vi "Information.vi"(8 "error in (no error)":errorcluster, 9 "Context":T1, 10 "Information":refnum<class "Information.lvclass">, 11 "Channel Scanner in":refnum<class "Channel Scanner.lvclass">) -> (0 "error out":errorcluster, 3 "Channel Scanner out":refnum<class "Channel Scanner.lvclass">)   [LabVIEW 2021, in "Channel Scanner.lvclass"]
uses:
  Channel Scanner.lvclass
  Publish-Subscribe/Interfaces/Information/Information.lvclass
  Publish-Subscribe/Context.ctl
  NHMFL_Core/Libraries/Instruments/Results/Acquired Result/Acquired Result.lvclass
  Channel Scanner.lvclass/Channel Scanner.ctl
  Read Channel scanner configuration.vi
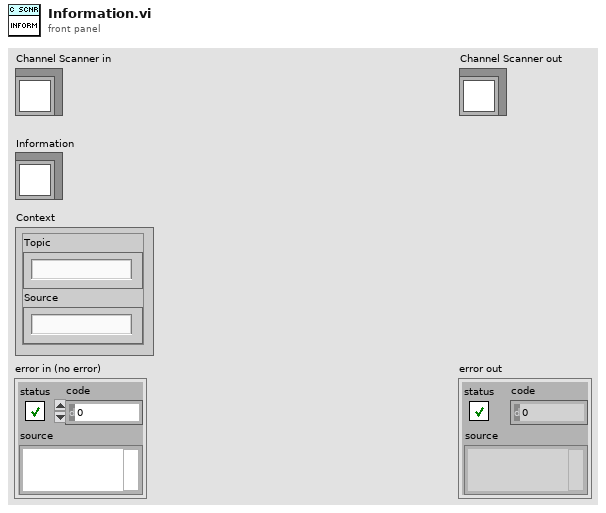
[diagram p1: front panel]
types:
  T1 = typedef "Context.ctl" = cluster{"Topic":string, "Source":string}
  T2 = typedef "Channel Scanner Configuration.ctl" = cluster{"Scan channels":i32[], "Group with measurement":string}
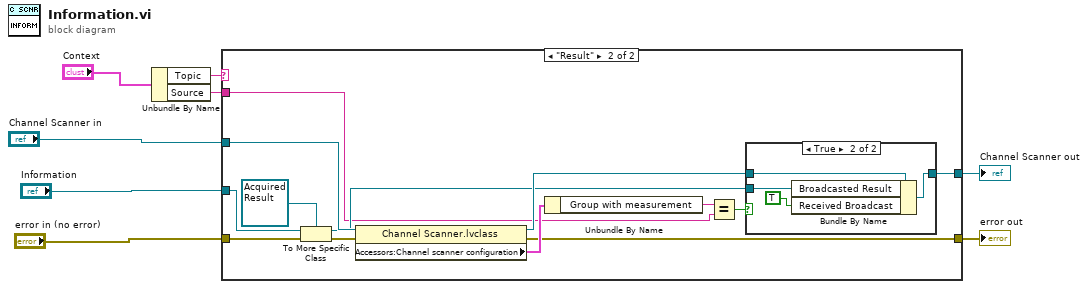
[diagram p0: block diagram]
diagram:
  n1 = Unbundle By Name("Context") -> ("Topic"=w8:string, "Source"=w3:string)
  n2 = case shown="\"Result\"" w8 {
    tunnel: "Information" -> [_ w22]
    tunnel: "error in (no error)" -> [w9 w21]
    tunnel: "Channel Scanner in" -> [w10 w16]
    tunnel: [w10 w12] -> w1
    tunnel: [w9 w13] -> w2
    tunnel: w3 -> [_ w11]
    frame "", Default {
    }
    frame "Result" {
      n3 = To More Specific Class(target class=refnum<class "Acquired Result.lvclass"> refnum ("Acquired Result.lvclass"), reference=w22, error in=w21) -> (specific class reference=w14:refnum<class "Acquired Result.lvclass">, error out=w15:errorcluster)
      n4 = property class="Channel Scanner.lvclass"(reference=w16, error in=w15) -> (reference out=w20:refnum<class "Channel Scanner.lvclass">, error out=w13:errorcluster, "Accessors:Channel scanner configuration"=w17:T2)
      n5 = Unbundle By Name(w17) -> ("Group with measurement"=w18:string)
      n6 = Equal?(x=w18, y=w11) -> (x = y?=w19:bool)
      n7 = case shown="True" w19 {
        tunnel: w20 -> [w24 w28]
        tunnel: [w24 w26] -> w12
        tunnel: w14 -> [_ w25]
        frame False {
        }
        frame True {
          n8 = Bundle By Name(cluster=w28, "Broadcasted Result"=w25, "Received Broadcast"=TRUE) -> (w26:refnum<class "Channel Scanner.lvclass">)
        }
      }
    }
  }
  "error out" <- w2
  "Channel Scanner out" <- w1
